vi "PSCHN_Para Define.vi"() -> (3 "PopUp Para":T3)   [LabVIEW 2016]
uses:
  Controls/PSCHN_Channel Para.ctl
panel:
  in  "Car*d":T2={"Module Type*"="", "Module Name*"="", "Used*?"=FALSE, "Sample Rate"=1000.0, "Channe*l"={"CHTag*"="", "Used?*"=FALSE, "CHName"="", "Unit"="MPa", "斜率"=0.0, "截距"=0.0}} caption="物理通道" {"Sample Rate" items=["100"=100.0, "200"=200.0, "500"=500.0, "1k"=1000.0, "2k"=2000.0, "5k"=5000.0, "10k"=10000.0, "20k"=20000.0, "40k"=40000.0]}
  # "带*号的不会在树形控件中显示"
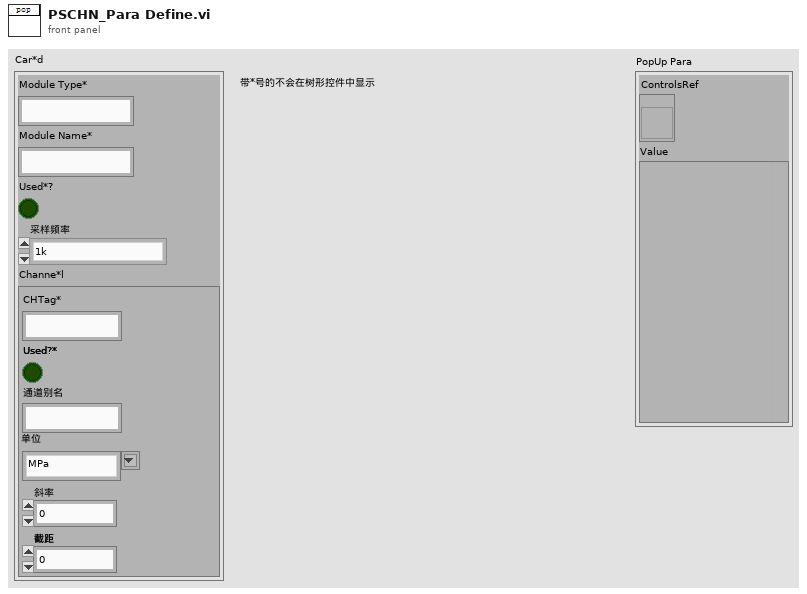
[diagram p1: front panel]
types:
  T1 = typedef "PSCHN_Channel Para.ctl" = cluster{"CHTag*":string, "Used?*":bool, "CHName":string, "Unit":string, "斜率":dbl, "截距":dbl}
  T2 = cluster{"Module Type*":string, "Module Name*":string, "Used*?":bool, "Sample Rate":dbl, "Channe*l":T1}
  T3 = cluster{"ControlsRef":refnum<vi>, "Value":variant}
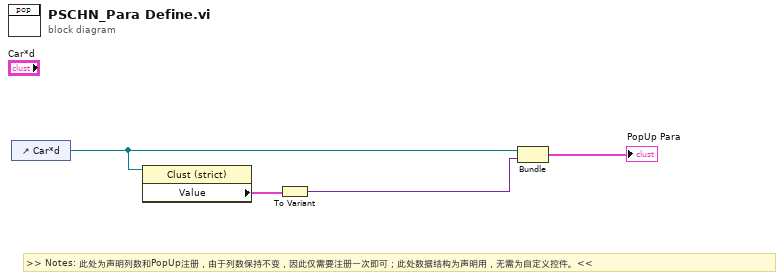
[diagram p0: block diagram]
diagram:
  # ">> Notes: 此处为声明列数和PopUp注册，由于列数保持不变，因此仅需要注册一次即可；此处数据结构为声明用，无需为自定义控件。<<"
  n1 = control-ref of="Car*d"() -> (w3:refnum<vi>)
  n2 = property class="Clust (strict)"(reference=w3) -> ("Value"=w4:T2)  [unwired: 1 in, 2 out]
  n3 = To Variant(anything=w4) -> (Variant=w2:variant)
  n4 = Bundle("Car*d"=w3, "Variant"=w2) -> (→"PopUp Para":cluster{"Car*d":refnum<vi>, "Variant":variant})  [unwired: 1 in]
